vi "Exercise 3-6.vi"() -> ()   [LabVIEW 2014]
panel:
  in  "stop":bool
  out "Fahrenheit":dbl
  out "Kelvin":dbl
  out "Celsius":dbl
  in  "Fahrenheit":dbl
  in  "Celsius":dbl
  # "To Do Farenheit, set Celcius to 0"
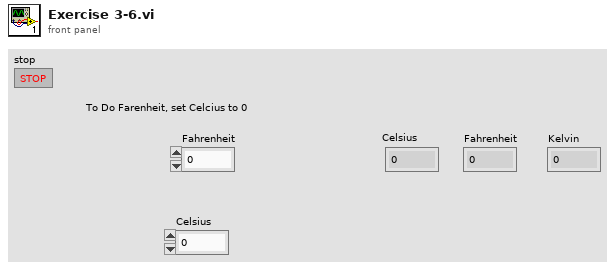
[diagram p1: front panel]
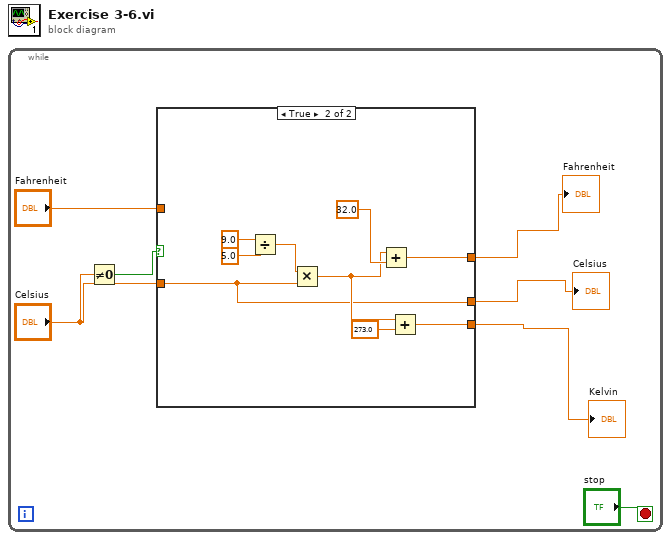
[diagram p0: block diagram]
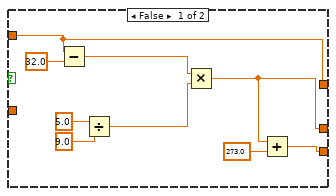
[diagram p2: hidden frame]
diagram:
  n1 = while {
    stop <- "stop" stop-if-true
    n2 = Not Equal To 0?(x="Celsius") -> (x != 0?=w4:bool)
    n3 = case shown="True" w4 {
      tunnel: [w14 w25] -> w7
      tunnel: [w10 w24] -> w6
      tunnel: "Fahrenheit" -> [w14 _]
      tunnel: [w9 w17] -> w1
      tunnel: "Celsius" -> [_ w17]
      frame False {
        n4 = Subtract(x=w14, y=32.0) -> (x-y=w15:dbl)
        n5 = Divide(x=5.0, y=9.0) -> (x/y=w16:dbl)
        n6 = Multiply(x=w15, y=w16) -> (x*y=w9:dbl)
        n7 = Add(x=w9, y=273.0) -> (x+y=w10:dbl)
      }
      frame True {
        n8 = Divide(x=9.0, y=5.0) -> (x/y=w18:dbl)
        n9 = Multiply(x=w18, y=w17) -> (x*y=w21:dbl)
        n10 = Add(x=w21, y=32.0) -> (x+y=w25:dbl)
        n11 = Add(x=w21, y=273.0) -> (x+y=w24:dbl)
      }
    }
    "Celsius" <- w1
    "Kelvin" <- w6
    "Fahrenheit" <- w7
  }
